vi "WRITETX.vi"(1 "Data to Write":u8[](array[numeric])=[0, 0, 0, 0, 0, 0, 0, 0] format="%x", 2 "Frames to Write":u8, 3 "Reg. Select":u8 format="%03b", 4 "SPI Config In":T1) -> (0 "SPI Config Out":T1)   [LabVIEW 2019]
uses:
  SPI/SPI Config.ctl
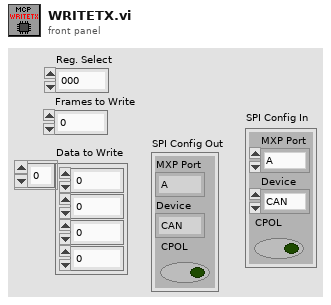
[diagram p1: front panel]
types:
  T1 = typedef "SPI Config.ctl" = cluster{"MXP Port":enum16{"A", "B"}, "Device":enum16{"CAN", "ENC", "IMU1", "IMU2"}, "CPOL":bool}
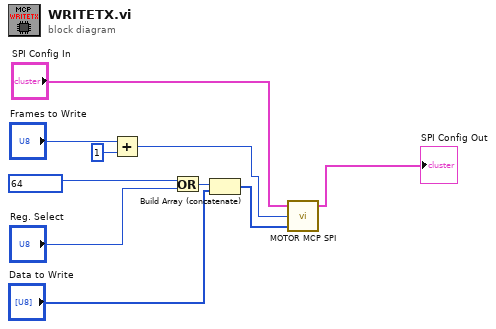
[diagram p0: block diagram]
diagram:
  n1 = Add(x="Frames to Write", y=u8 1) -> (x+y=w2:u8)
  n2 = Or(x=u8 64, y="Reg. Select") -> (x .or. y?=w9:u8)
  n3 = Build Array (concatenate)(w9, "Data to Write") -> (w1:u8[])
  n4 = call "MOTOR MCP SPI.vi"("Data to Write"=w1, "Frames to Write"=w2, "SPI Config In"="SPI Config In") -> ("SPI Config Out"=→"SPI Config Out":T1)  [unwired: 2 out]
